vi "Get MLJ Max Stage Acceleration.vi"(8 "error in (no error)":errorcluster, 10 "Cluster in":T1, 11 "MLJ Reference In":refnum<k24>) -> (0 "error out":errorcluster, 2 "Cluster out":T1, 3 "MLJ Reference Out":refnum<k24>)   [LabVIEW 2018]
uses:
  Controls/Translation Stage Cluster.ctl
  General/Controls/Translation Stage Types.ctl
  C:/Project/SSOCT/Labview Software/Thorlabs.MotionControl.Controls.dll
  Thorlabs.MotionControl.Controls.dll
  C:/Project/SSOCT/Labview Software/Thorlabs.MotionControl.IntegratedStepperMotorsCLI.dll
  Thorlabs.MotionControl.IntegratedStepperMotorsCLI.dll
  C:/Project/SSOCT/Labview Software/Thorlabs.MotionControl.GenericMotorCLI.dll
  Thorlabs.MotionControl.GenericMotorCLI.dll
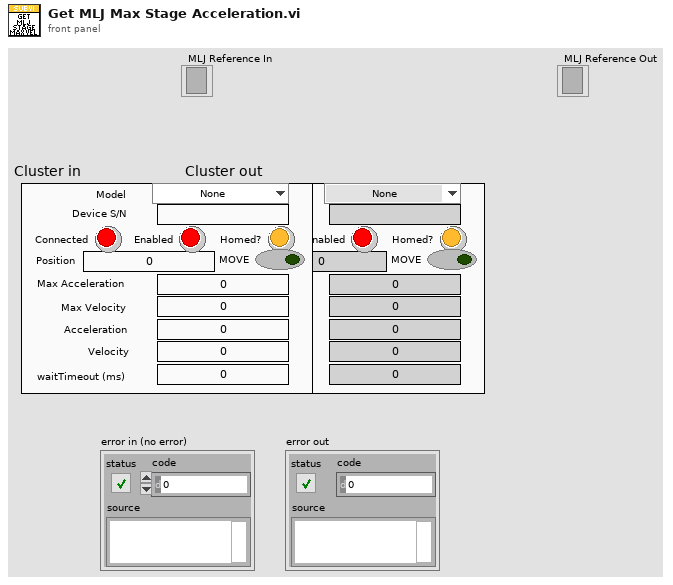
[diagram p1: front panel]
types:
  T1 = typedef "Translation Stage Cluster.ctl" = cluster{"Position":dbl, "Is.Enabled?":bool, "Is.Connected?":bool, "Device SN":string, "AccelerationMaximum":dbl, "VelocityMaximum":dbl, "Acceleration":dbl, "Velocity":dbl, "waitTimeout (ms)":i32, "Model":T2, "Is.Homed?":bool, "MOVE":bool}
  T2 = typedef "Translation Stage Types.ctl" = enum16{"None", "Thorlabs LTS", "Thorlabs MLJ"}
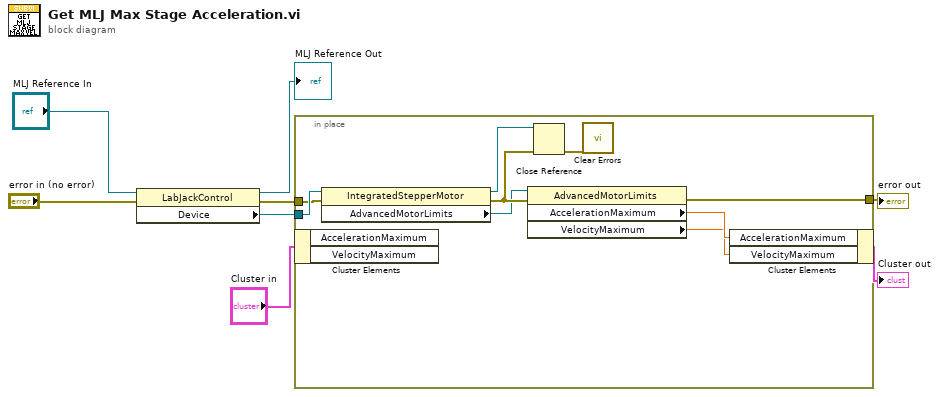
[diagram p0: block diagram]
diagram:
  n1 = property class="LabJackControl"(reference="MLJ Reference In", error in="error in (no error)") -> (reference out=→"MLJ Reference Out":refnum<k24>, error out=w4:errorcluster, "Device"=w2:refnum<k24>)
  n2 = in-place {
    in-place-border: w4 -> [w16]
    in-place-border: w2 -> [w17]
    in-place-border: [w10] -> w1
    n3 = in-place-cluster #1("Cluster in") -> ()  [unwired: 2 out]
    n4 = property class="IntegratedStepperMotor"(reference=w17, error in=w16) -> (reference out=w15:refnum<k24>, error out=w14:errorcluster, "AdvancedMotorLimits"=w13:refnum<k24>)
    n5 = property class="AdvancedMotorLimits"(reference=w13, error in=w14) -> (error out=w10:errorcluster, "AccelerationMaximum"=w12:dbl, "VelocityMaximum"=w11:dbl)  [unwired: 1 out]
    n6 = Close Reference(reference=w15, error in (no error)=w14) -> (error out=w9:errorcluster)
    n7 = call <vilib>:"Clear Errors.vi"("error in (no error)"=w9) -> ()  [unwired: 5 in, 2 out]
    n8 = in-place-cluster #1("AccelerationMaximum"=w12, "VelocityMaximum"=w11) -> (→"Cluster out":T1)
  }
  "error out" <- w1
